vi "Check Pattern Name.vi"(8 "error in (no error)":errorcluster, 10 "SPI FRM Config in":T1[](array[typedef]) {"Addr" format="%x"; "Data" format="%x"}, 11 "Path":path) -> (0 "error out":errorcluster, 2 "SPI FRM Config out":T1[](array[typedef]) {"Addr" format="%x"; "Data" format="%x"})   [LabVIEW 2018, in "Config_Read_SPI.lvclass"]
uses:
  Config_Read_SPI.lvclass
  SPI_FRM_Config.ctl
  Classes/Config_Read/RW_Option.ctl
  SPI_Mode.ctl
  Classes/Config_Read/Config_Read_BML.lvclass
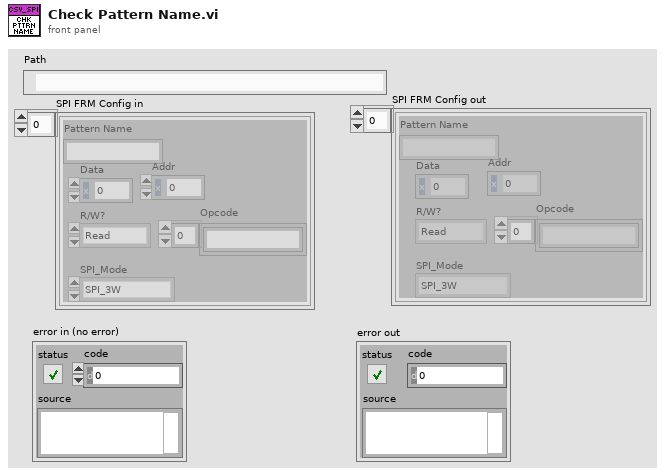
[diagram p1: front panel]
types:
  T1 = typedef "Config_Read_SPI.lvclass/SPI_FRM_Config.ctl" = cluster{"Pattern Name":string, "Data":u16, "Addr":u16, "R/W?":T2, "Opcode":string[], "SPI_Mode":T3}
  T2 = typedef "Config_Read_BML.lvclass/RW_Option.ctl" = enum16{"Read", "Write", "R/W"}
  T3 = typedef "Config_Read_SPI.lvclass/SPI_Mode.ctl" = enum16{"SPI_3W", "SPI_4W"}
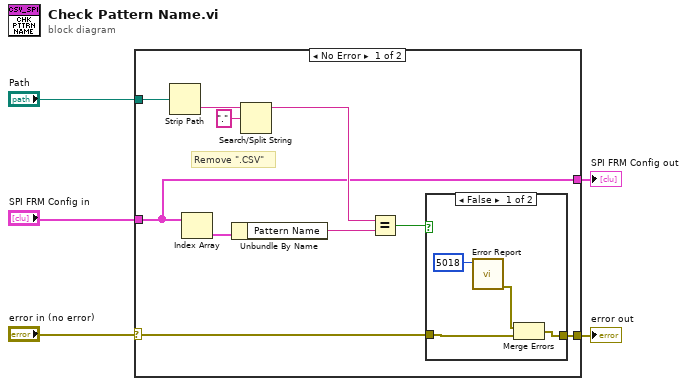
[diagram p0: block diagram]
diagram:
  n1 = case shown="No Error" "error in (no error)" {
    selector: "error in (no error)" -> [w11 w21]
    tunnel: "SPI FRM Config in" -> [w6 _]
    tunnel: "Path" -> [w15 _]
    tunnel: [w10 w21] -> w3
    tunnel: [w6 _] -> w1
    frame No Error {
      # "Remove \".CSV\""
      n2 = Strip Path(path=w15) -> (name=w9:string)  [unwired: 1 out]
      n3 = Index Array(array=w6) -> (element=w14:T1)  [unwired: 1 in]
      n4 = Unbundle By Name(w14) -> ("Pattern Name"=w13:string)
      n5 = Search/Split String(string=w9, search string/char (-)=".") -> (substring before match=w7:string)  [unwired: 1 in, 2 out]
      n6 = Equal?(x=w7, y=w13) -> (x = y?=w12:bool)
      n7 = case shown="False" w12 {
        tunnel: w11 -> [w17 w20]
        tunnel: [w16 w20] -> w10
        frame False {
          n8 = call "Error Report.vi"("Error Code"=i16 5018) -> ("error out"=w18:errorcluster)  [unwired: 10 in]
          n9 = Merge Errors(w18, w17) -> (w16:errorcluster)
        }
        frame True {
        }
      }
    }
    frame Error {
    }
  }
  "error out" <- w3
  "SPI FRM Config out" <- w1
